vi "保存mes.vi"(11 "参数值":T1(array[cluster])) -> (0 "error out":errorcluster, 3 "出站成功":bool)   [LabVIEW 2020]
uses:
  Global.vi
  <vilib>/Utility/file.llb/Write Delimited Spreadsheet (string).vi
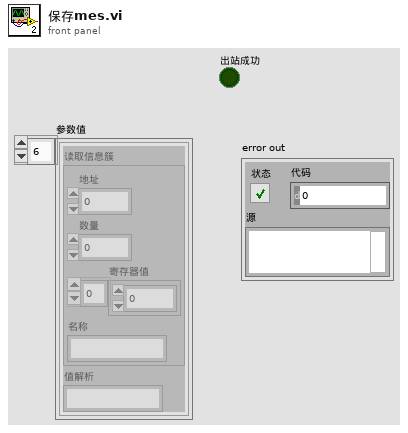
[diagram p1: front panel]
types:
  T1 = cluster{"读取信息簇":cluster{"地址":u16, "数量":u16, "寄存器值":u16[], "名称":string}, "值解析":string}[]
  T2 = cluster{"Server":string, "audit_mode":string, "tsid":string, "model":string, "product":string, "test_station":string, "station_id":string, "test_station_name":string, "Webservice":string}
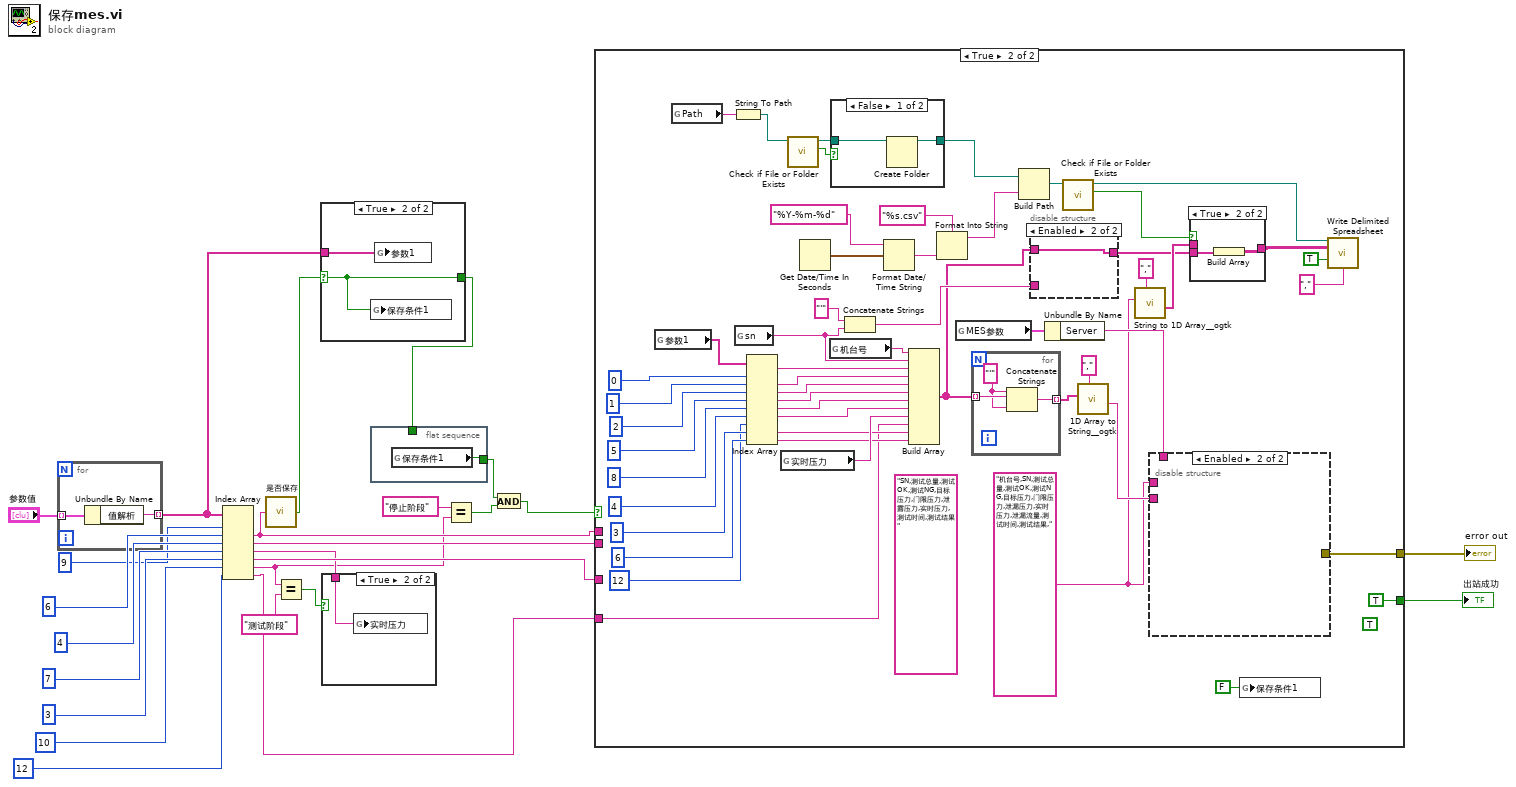
[diagram p0: block diagram]
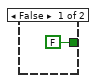
[diagram p4: hidden frame]
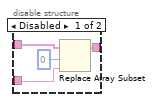
[diagram p5: hidden frame]
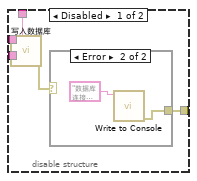
[diagram p6: hidden frame]
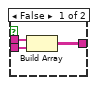
[diagram p8: hidden frame]
diagram:
  n1 = for {
    tunnel: "参数值" -> [w27] mode=indexing
    tunnel: [w26] -> w9 mode=indexing
    n2 = Unbundle By Name(w27) -> ("值解析"=w26:string)
  }
  n3 = Index Array(array=w9, index #1=9 ("索引"), index #2=6 ("索引"), index #3=4 ("索引"), index #4=7 ("索引"), index #5=3 ("索引"), index #6=10 ("索引"), index #7=12 ("索引")) -> (element #2=w20:string, element #3=w19:string, element #4=w13:string, element #5=w18:string, element #6=w8:string, element #7=w5:string)  [unwired: 1 out]
  n4 = call "是否保存.vi"("测试结果"=w20) -> ("保存"=w10:bool)
  n5 = Equal?(x=w8, y="测试阶段") -> (x = y?=w14:bool)
  n6 = case shown="True" w10 {
    selector: w10 -> [w28 w29]
    tunnel: w9 -> [_ w30]
    tunnel: [w28 w29] -> w1
    frame False {
    }
    frame True {
      n7 = global write "Global.vi" "保存条件1"(w29) -> ()
      n8 = global write "Global.vi" "参数1"(w30) -> ()
    }
  }
  n9 = case shown="True" w14 {
    tunnel: w13 -> [_ w31]
    frame False {
    }
    frame True {
      n10 = global write "Global.vi" "实时压力"(w31) -> ()
    }
  }
  n11 = flat-sequence {
    tunnel: [w32] -> w2
    tunnel: w1 -> [_]
    frame #0 {
      n12 = global read "Global.vi" "保存条件1"() -> (w32:bool)
    }
  }
  n13 = Equal?(x="停止阶段" ("y"), y=w8) -> (x = y?=w4:bool)
  n14 = And(x=w2, y=w4) -> (x .and. y?=w3:bool)
  n15 = case shown="True" w3 {
    tunnel: w20 -> [_ _]
    tunnel: w19 -> [_ _]
    tunnel: w18 -> [_ _]
    tunnel: [_ w70] -> w12
    tunnel: [FALSE TRUE] -> w11
    tunnel: w5 -> [_ w37]
    frame False {
    }
    frame True {
      (unwired) "SN,测试总量,测试OK,测试NG,目标压力,门限压力,泄露压力,实时压力,测试时间,测试结果" ("测量项目")
      (unwired) TRUE
      w44 = "机台号,SN,测试总量,测试OK,测试NG,目标压力,门限压力,泄漏压力,实时压力,泄漏流量,测试时间,测试结果," ("测量项目")
      n16 = global read "Global.vi" "参数1"() -> (w36:string[])
      n17 = global read "Global.vi" "Path"() -> (w59:string)
      n18 = String To Path(string=w59) -> (path=w58:path)
      n19 = global read "Global.vi" "sn"() -> (w48:string)
      n20 = Index Array(array=w36, index #1=0 ("索引"), index #2=1 ("索引"), index #3=2 ("索引"), index #4=5 ("索引"), index #5=8 ("索引"), index #6=4 ("索引"), index #7=12 ("索引"), index #8=3 ("索引"), index #9=6 ("索引")) -> (element #1=w80:string, element #2=w79:string, element #3=w78:string, element #4=w77:string, element #5=w76:string, element #6=w75:string, element #8=w39:string, element #9=w40:string)  [unwired: 1 out]
      n21 = global read "Global.vi" "实时压力"() -> (w74:string)
      n22 = call <vilib>:"Check if File or Folder Exists.vi"("path"=w58) -> ("file or folder exists?"=w63:bool, "dup path"=w62:path)  [unwired: 8 in, 1 out]
      n23 = Get Date/Time In Seconds() -> (seconds since 1Jan1904=w66:timestamp)
      n24 = global read "Global.vi" "机台号"() -> (w34:string)
      n25 = case shown="False" w63 {
        tunnel: w62 -> [w106 w107]
        tunnel: [w105 w107] -> w61
        frame False {
          n26 = Create Folder(path (use dialog)=w106) -> (created path=w105:path)  [unwired: 2 in, 2 out]
        }
        frame True {
        }
      }
      n27 = Concatenate Strings("'", w48) -> (w47:string)
      n28 = Format Date/Time String(time format string (%c)="%Y-%m-%d" ("时间格式字符串(%c)"), seconds (now)=w66) -> (date/time string=w65:string)  [unwired: 1 in]
      n29 = Build Array(w34, w48, w80, w79, w78, w77, w76, w75, w74, w37, w39, w40) -> (w45:string[])
      n30 = Format Into String(format string="%s.csv" ("格式字符串"), w65) -> (resulting string=w64:string)  [unwired: 2 in, 1 out]
      n31 = global read "Global.vi" "MES参数"() -> (w68:T2)
      n32 = for {
        tunnel: w45 -> [w110] mode=indexing
        tunnel: [w108] -> w72 mode=indexing
        w109 = "'"
        n33 = Concatenate Strings(w109, w110, w109) -> (w108:string)
      }
      n34 = Build Path(base path=w61, name or relative path=w64) -> (appended path=w60:path)
      n35 = disable-structure shown="Enabled" {
        disable-tunnel: w47 -> [w89 _]
        disable-tunnel: [w88 w91] -> w46
        disable-tunnel: w45 -> [w87 w91]
        frame Disabled {
          n36 = Replace Array Subset(array=w87, new element=w89, index=0) -> (w88:string[])
        }
        frame Enabled {
        }
      }
      n37 = Unbundle By Name(w68) -> ("Server"=w67:string)
      n38 = call <vilib>:"Check if File or Folder Exists.vi"("path"=w60) -> ("file or folder exists?"=w57:bool, "dup path"=w49:path)  [unwired: 8 in, 1 out]
      n39 = call <userlib>:"1D Array to String__ogtk.vi"("delimiter (Tab)"=",", "Array of Strings"=w72) -> ("delimited string"=w71:string)  [unwired: 9 in]
      n40 = call <userlib>:"String to 1D Array__ogtk.vi"("delimiter (Tab)"=",", "string"=w44) -> ("Array of Strings"=w53:string[])  [unwired: 9 in]
      n41 = disable-structure shown="Enabled" {
        disable-tunnel: w71 -> [w96 _]
        disable-tunnel: [w94 _] -> w70
        disable-tunnel: w67 -> [w93 _]
        disable-tunnel: w44 -> [w92 _]
        frame Disabled {
          n42 = call "写入数据库.vi"("SERVER(IP)"=w93, "values"=w96, "测试项目"=w92) -> ("error out"=w95:errorcluster)  [unwired: 8 in]
          n43 = case shown="Error" w95 {
            selector: w95 -> [w97 _]
            tunnel: [w97 w98] -> w94
            frame No Error {
            }
            frame Error {
              n44 = call "Write to Console.vi"("Input"="数据库连接错误。" ("消息")) -> ("error out"=w98:errorcluster)  [unwired: 10 in]
            }
          }
        }
        frame Enabled {
        }
      }
      n45 = case shown="True" w57 {
        tunnel: w53 -> [w102 _]
        tunnel: w46 -> [w101 w104]
        tunnel: [w100 w103] -> w50
        frame False {
          n46 = Build Array(w102, w101) -> (w100:string[][])
        }
        frame True {
          n47 = Build Array(w104) -> (w103:string[][])
        }
      }
      n48 = global write "Global.vi" "保存条件1"(FALSE ("保存条件1")) -> ()
      n49 = call-poly <vilib>:"Write Delimited Spreadsheet.vi"("file path (dialog if empty)"=w49, "2D data"=w50, "append to file? (new file:F)"=TRUE ("append to file? (F)"), "delimiter (\\t)"="," ("delimiter (\\t)")) -> ()  [unwired: 10 in, 2 out]
    }
  }
  "出站成功" <- w11
  "error out" <- w12
